vi "send_pwm.vi"(8 "error in (no error)":errorcluster, 9 "streaming":i32, 10 "packet":T1, 11 "handle":u64) -> (0 "error out":errorcluster, 1 "function return":i32)   [LabVIEW 2017, in "buddy.lvlib"]
doc: "EXPORT int buddy_send_dac(hid_device *handle, general_packet_t *packet, bool streaming);"
uses:
  buddy.lvlib
  buddy_x64.dll
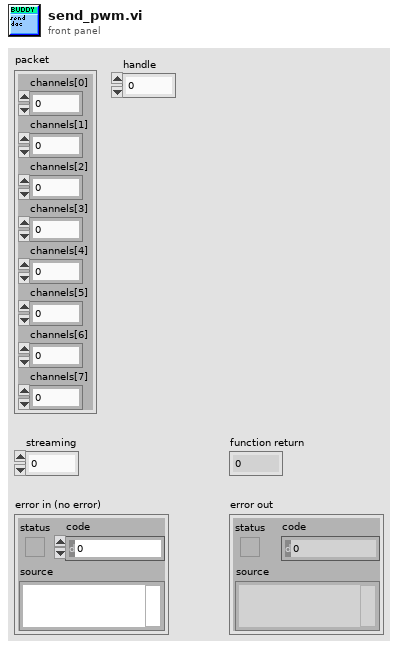
[diagram p1: front panel]
types:
  T1 = cluster{"channels[0]":u32, "channels[1]":u32, "channels[2]":u32, "channels[3]":u32, "channels[4]":u32, "channels[5]":u32, "channels[6]":u32, "channels[7]":u32}
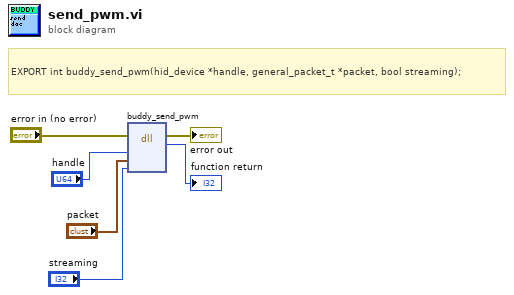
[diagram p0: block diagram]
diagram:
  # "EXPORT int buddy_send_pwm(hid_device *handle, general_packet_t *packet, bool streaming);"
  n1 = dll-call lib="C:/Users/shraken/shraken_code/usbhid_buddy/lib/libbuddy/bindings/labview/utility_vi/buddy_x64.dll" fn="buddy_send_pwm"(error in="error in (no error)", "handle"="handle", "packet"="packet", "streaming"="streaming") -> (error out=→"error out":errorcluster, "return type"=→"function return":i32)  [unwired: 5 in, 1 out]
